vi "Benchmark SV Receive LV2012 - NI Verified - 2.vi"() -> ()   [LabVIEW 2015]
panel:
  out "data out":T1
  in  "stop":bool
  # "Overview:  Coding that exemplifies how to benchmark the communication of Shared Variables.\nRequirements: LabVIEW 2012 or compatible\nInstructions:\n1. Run this VI\n2. Watch the amount of time it takes to communicate on the \"Benchmark SV Send  LV2012 - NI Verified.vi\" \n3. Stop both VIs"
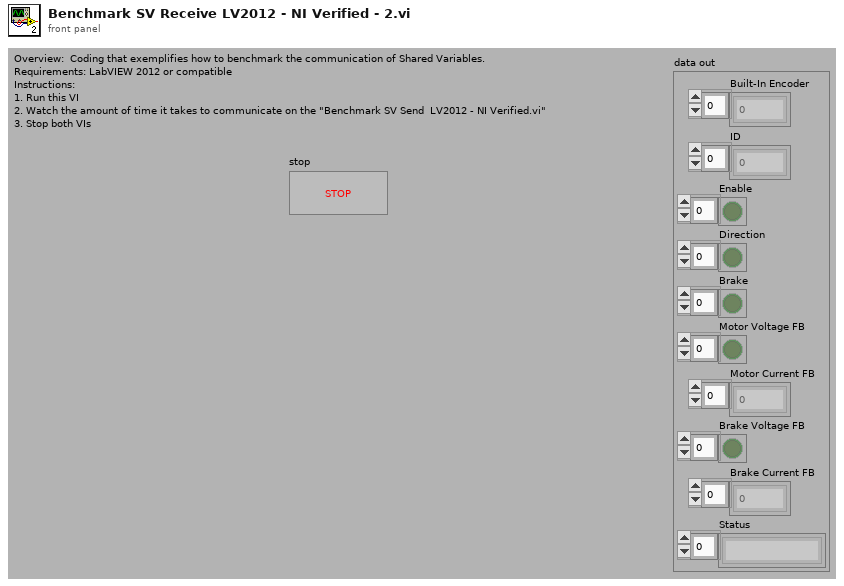
[diagram p1: front panel]
types:
  T1 = cluster{"Built-In Encoder":i32[], "ID":i16[], "Enable":bool[], "Direction":bool[], "Brake":bool[], "Motor Voltage FB":bool[], "Motor Current FB":i32[], "Brake Voltage FB":bool[], "Brake Current FB":i32[], "Status":string[]}
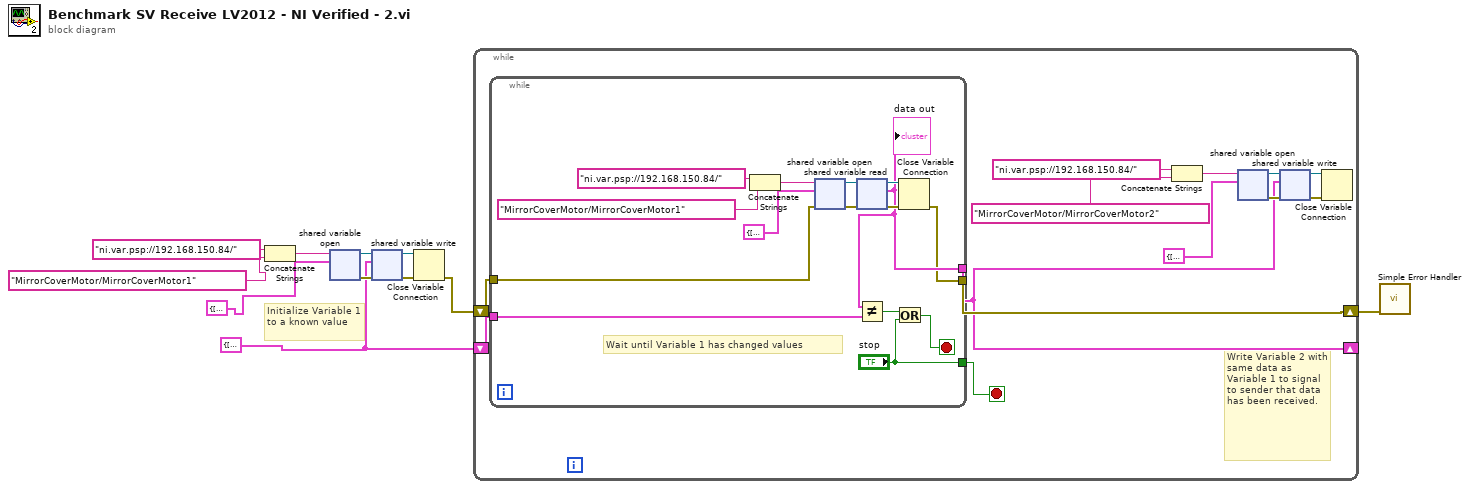
[diagram p0: block diagram]
diagram:
  w1 = T1 {"Built-In Encoder"=[], "ID"=[], "Enable"=[], "Direction"=[], "Brake"=[], "Motor Voltage FB"=[], "Motor Current FB"=[], "Brake Voltage FB"=[], "Brake Current FB"=[], "Status"=[]} ("input cluster")
  # "Initialize Variable 1 to a known value"
  n1 = Concatenate Strings("ni.var.psp://192.168.150.84/" ("string"), "MirrorCoverMotor/MirrorCoverMotor1") -> (w10:string)
  n2 = shared-variable-open(w10, T1 {"Built-In Encoder"=[], "ID"=[], "Enable"=[], "Direction"=[], "Brake"=[], "Motor Voltage FB"=[], "Motor Current FB"=[], "Brake Voltage FB"=[], "Brake Current FB"=[], "Status"=[]} ("MirrorCoverMotor")) -> (w8:refnum<k21>, w6:errorcluster)  [unwired: 2 in]
  n3 = shared-variable-write(w8, w6, w1) -> (w7:refnum<k21>, w5:errorcluster)
  n4 = Close Variable Connection(8:w5, 11:w7) -> (0:w4:errorcluster)
  n5 = while {
    shift-right: [w14] -> _
    shift-left: w1 -> [w24]
    shift-right: [w21] -> w11
    shift-left: w4 -> [w22]
    stop <- w23 stop-if-true
    # "Write Variable 2 with same data as Variable 1 to signal to sender that data has been received."
    n6 = while {
      tunnel: w24 -> [w39]
      tunnel: [w29] -> w14
      tunnel: ["stop"] -> w23
      tunnel: [w28] -> w21
      tunnel: w22 -> [w27]
      stop <- w36 stop-if-true
      # "Wait until Variable 1 has changed values"
      n7 = Concatenate Strings("ni.var.psp://192.168.150.84/" ("string"), "MirrorCoverMotor/MirrorCoverMotor1") -> (w34:string)
      n8 = shared-variable-open(w34, w27, T1 {"Built-In Encoder"=[], "ID"=[], "Enable"=[], "Direction"=[], "Brake"=[], "Motor Voltage FB"=[], "Motor Current FB"=[], "Brake Voltage FB"=[], "Brake Current FB"=[], "Status"=[]} ("MirrorCoverMotor")) -> (w33:refnum<k21>, w32:errorcluster)  [unwired: 1 in]
      n9 = shared-variable-read(w33, w32) -> (w31:refnum<k21>, w30:errorcluster, w29:T1)  [unwired: 1 out]
      "data out" <- w29
      n10 = Not Equal?(x=w29, y=w39) -> (x != y?=w38:bool)
      n11 = Or(x=w38, y="stop") -> (x .or. y?=w36:bool)
      n12 = Close Variable Connection(8:w30, 11:w31) -> (0:w28:errorcluster)
    }
    n13 = Concatenate Strings("ni.var.psp://192.168.150.84/" ("string"), "MirrorCoverMotor/MirrorCoverMotor2") -> (w19:string)
    n14 = shared-variable-open(w19, T1 {"Built-In Encoder"=[], "ID"=[], "Enable"=[], "Direction"=[], "Brake"=[], "Motor Voltage FB"=[], "Motor Current FB"=[], "Brake Voltage FB"=[], "Brake Current FB"=[], "Status"=[]} ("MirrorCoverMotor")) -> (w18:refnum<k21>, w17:errorcluster)  [unwired: 2 in]
    n15 = shared-variable-write(w18, w17, w14) -> (w16:refnum<k21>, w15:errorcluster)
    n16 = Close Variable Connection(8:w15, 11:w16) -> ()  [unwired: 1 out]
  }
  n17 = call <vilib>:"Simple Error Handler.vi"("error in (no error)"=w11) -> ()  [unwired: 4 in, 5 out]
